vi "Initialize.vi"(7 "Path":path, 8 "error in (no error)":errorcluster, 9 "Invoked from wizard":bool, 10 "Object":T2, 11 "Class in":refnum<class "AB_UI_Frmwk_Installer.lvclass">) -> (0 "error out":errorcluster, 1 "helpTopics out":string[](array[string]), 2 "pageTitles out":string[](array[string]), 3 "Class out":refnum<class "AB_UI_Frmwk_Installer.lvclass">, 4 "helpFile":string, 5 "pageMsgData":T1[](array[typedef]))   [LabVIEW 2020, in "AB_UI_Frmwk_Installer.lvclass"]
uses:
  <vilib>/AppBuilder/IB_Classes/Installer/UI/AB_UI_Frmwk_Installer.lvclass
  <vilib>/AppBuilder/IB_Classes/Installer/UI/AB_UI_Frmwk_Installer.lvclass/AB_UI_Frmwk_Installer.ctl
  <resource>/Framework/Providers/Builds/AppBuilder/AB_UI_Framework_MsgToPage_Action.ctl
  <resource>/Framework/Providers/Builds/AppBuilder/AB_UI_Page_MessageData.ctl
  <vilib>/AppBuilder/IB_Classes/Installer/Installer.lvclass
  <resource>/Framework/Providers/Builds/Installer/SRdB/IB_SRdB_Action.ctl
  <resource>/Framework/Providers/Builds/Installer/SRdB_Proj/SRdB_Proj_Action.ctl
  <resource>/Framework/Providers/Builds/Installer/SRdb_Bld/SRdB_Bld_action.ctl
  <resource>/Framework/Providers/Builds/Installer/SRdB_Icon/SRdB_Icon_action.ctl
  AppLibs/distkit/MDF/NI_MDF.lvlib
  <resource>/Framework/Providers/Builds/Installer/CDK_GLOBAL_STRINGS.vi
  <resource>/Framework/Providers/API/ItemRef.ctl
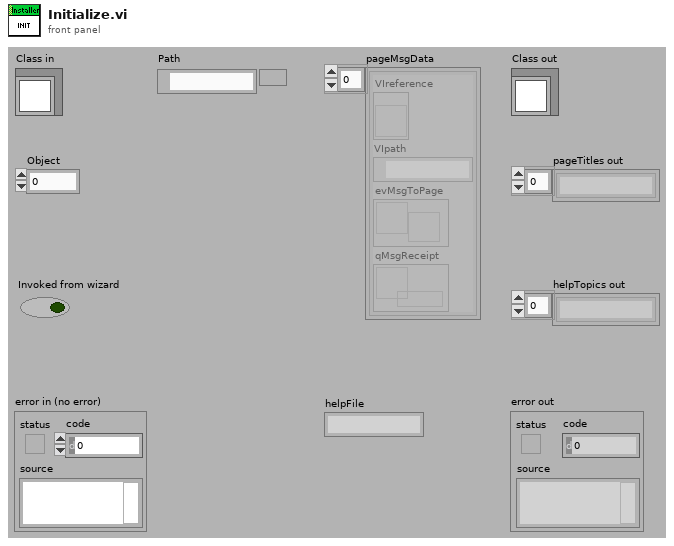
[diagram p1: front panel]
types:
  T1 = typedef "AB_UI_Page_MessageData.ctl" = cluster{"VIreference":refnum<vi>, "VIpath":path, "evMsgToPage":refnum<user-event>, "qMsgReceipt":refnum<queue>}
  T2 = typedef "ItemRef.ctl" = u64
  T3 = typedef "SRdB_Icon_action.ctl" = enum16{"read", "write", "create", "delete", "initialize", "unInitialize", "getLock", "readAll", "writeAll"}
  T4 = typedef "SRdB_Bld_action.ctl" = enum16{"read", "write", "create", "delete", "initialize", "unInitialize", "getLock", "readAll", "writeAll"}
  T5 = typedef "IB_SRdB_Action.ctl" = enum16{"read", "write", "create", "delete", "initialize", "unInitialize", "getLock", "readAll", "writeAll"}
  T6 = typedef "SRdB_Proj_Action.ctl" = enum16{"read", "write", "create", "delete", "initialize", "unInitialize", "getLock", "readAll", "writeAll"}
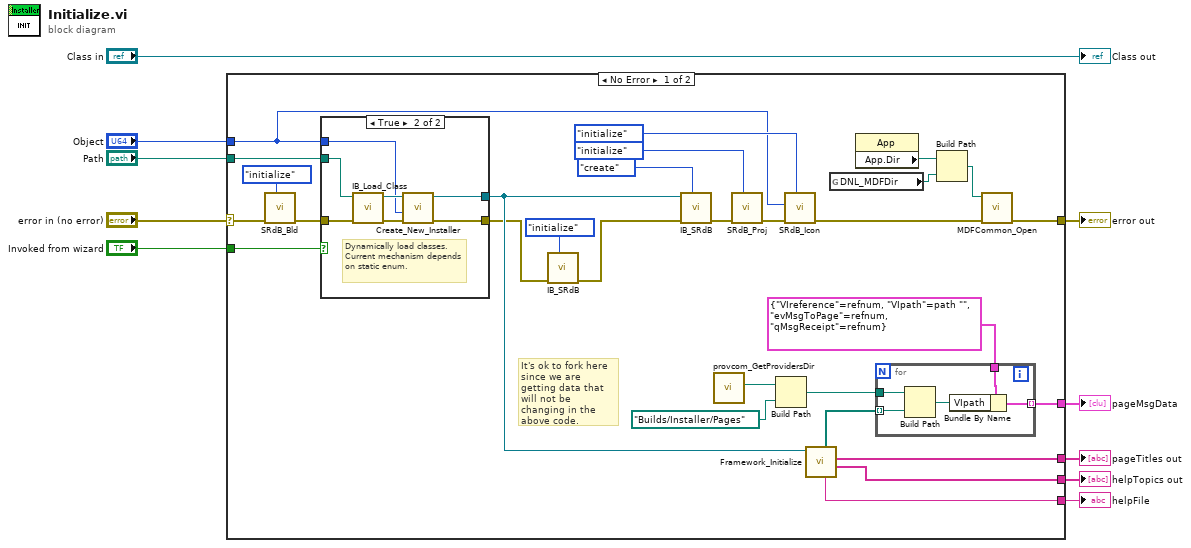
[diagram p0: block diagram]
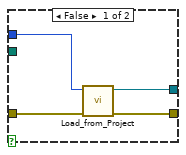
[diagram p2: hidden frame]
diagram:
  n1 = case shown="No Error" "error in (no error)" {
    selector: "error in (no error)" -> [w20 w56]
    tunnel: "Object" -> [w16 _]
    tunnel: [w11 w56] -> w5
    tunnel: [w37 _] -> w4
    tunnel: "Invoked from wizard" -> [w36 _]
    tunnel: [w30 _] -> w2
    tunnel: [w31 _] -> w1
    tunnel: [w29 _] -> w3
    tunnel: "Path" -> [w34 _]
    frame No Error {
      # "It's ok to fork here since we are getting data that will not be changing in the above code."
      n2 = call <resource>:"SRdB_Bld.vi"("action"=SRdB_Bld_action."initialize", "error in (no error)"=w20) -> ("error out"=w19:errorcluster)  [unwired: 1 in, 8 out]
      n3 = case shown="True" w36 {
        tunnel: [w41 w45] -> w27
        tunnel: w19 -> [w40 w50]
        tunnel: w16 -> [w43 w44]
        tunnel: [w42 w46] -> w28
        tunnel: w34 -> [_ w49]
        frame False {
          n4 = call <vilib>:"Load_from_Project.vi"("error in (no error)"=w40, "Object"=w43) -> ("error out"=w41:errorcluster, "Installer out"=w42:refnum<class "Installer.lvclass">)  [unwired: 2 in, 6 out]
        }
        frame True {
          # "Dynamically load classes. Current mechanism depends on static enum."
          n5 = call <vilib>:"IB_Load_Class.vi"("error in (no error)"=w50, "IB_Class path"=w49) -> ("error out"=w48:errorcluster, "IB_Installer out"=w47:refnum<class "Installer.lvclass">)  [unwired: 8 out]
          n6 = call-dynamic "Create_New_Installer.vi"("error in (no error)"=w48, "buildObject"=w44, "Class in"=w47) -> ("error out"=w45:errorcluster, "Class out"=w46:refnum<class "Installer.lvclass">)  [unwired: 3 in, 4 out]
        }
      }
      n7 = call <resource>:"IB_SRdB.vi"("action"=IB_SRdB_Action."initialize", "error in (no error)"=w27) -> ("error out"=w26:errorcluster)  [unwired: 1 in, 8 out]
      n8 = call <resource>:"IB_SRdB.vi"("action"=IB_SRdB_Action."create", "error in (no error)"=w26, "data in"=w28) -> ("error out"=w24:errorcluster)  [unwired: 8 out]
      n9 = call <resource>:"provcom_GetProvidersDir.vi"() -> ("projProv Dir"=w33:path)  [unwired: 11 out]
      n10 = call <resource>:"SRdB_Proj.vi"("action"=SRdB_Proj_Action."initialize", "error in (no error)"=w24) -> ("error out"=w17:errorcluster)  [unwired: 1 in, 8 out]
      n11 = Build Path(base path=w33, name or relative path=path "Builds/Installer/Pages") -> (appended path=w38:path)
      n12 = call <resource>:"SRdB_Icon.vi"("action"=SRdB_Icon_action."initialize", "error in (no error)"=w17, "Object"=w16) -> ("error out"=w12:errorcluster)  [unwired: 1 in, 7 out]
      n13 = call-dynamic "Framework_Initialize.vi"("Class in"=w28) -> ("helpTopics"=w30:string[], "pageTitles"=w29:string[], "helpFile"=w31:string, "pages"=w32:path[])  [unwired: 1 in, 6 out]
      n14 = global read "CDK_GLOBAL_STRINGS.vi" "DNL_MDFDir"() -> (w14:path)
      n15 = property class="App"() -> ("App.Dir"=w15:path)  [unwired: 2 in, 2 out]
      n16 = for {
        tunnel: w38 -> [w55]
        tunnel: [w51] -> w37 mode=indexing
        tunnel: T1 {"VIreference"=refnum, "VIpath"=path "", "evMsgToPage"=refnum, "qMsgReceipt"=refnum} ("qPageMsgs") -> [w53]
        tunnel: w32 -> [w54] mode=indexing
        n17 = Build Path(base path=w55, name or relative path=w54) -> (appended path=w52:path)
        n18 = Bundle By Name(cluster=w53, "VIpath"=w52) -> (w51:T1)
      }
      n19 = Build Path(base path=w15, name or relative path=w14) -> (appended path=w13:path)
      n20 = call "MDFCommon_Open.vi"("error in (no error)"=w12, "redist directory"=w13) -> ("error out"=w11:errorcluster)  [unwired: 9 in]
    }
    frame Error {
    }
  }
  "error out" <- w5
  "pageMsgData" <- w4
  "pageTitles out" <- w3
  "helpTopics out" <- w2
  "helpFile" <- w1
  "Class out" <- "Class in"
